vi "SafeBiasSet.vi"(0 "Application ref in":refnum<vi>, 1 "Bias (V)":sgl=-2.0 format="%_5p", 2 "Ramp":bool=TRUE, 3 "error in (no error)":errorcluster, 4 "milliseconds to wait":u32=2) -> (7 "Application ref out":refnum<vi>, 10 "Error out":errorcluster)   [LabVIEW 2021]
uses:
  <userlib>/Nanonis Prog Interface V5/Nanonis Prog Interface.lvlib
panel:
  in  "Bias (V) StepSize":sgl=0.05 format="%_5p"
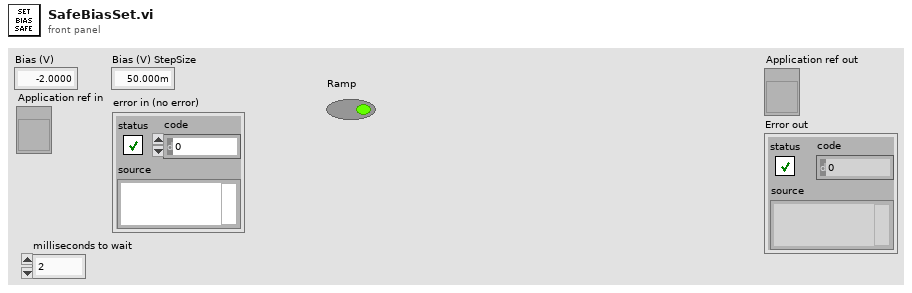
[diagram p1: front panel]
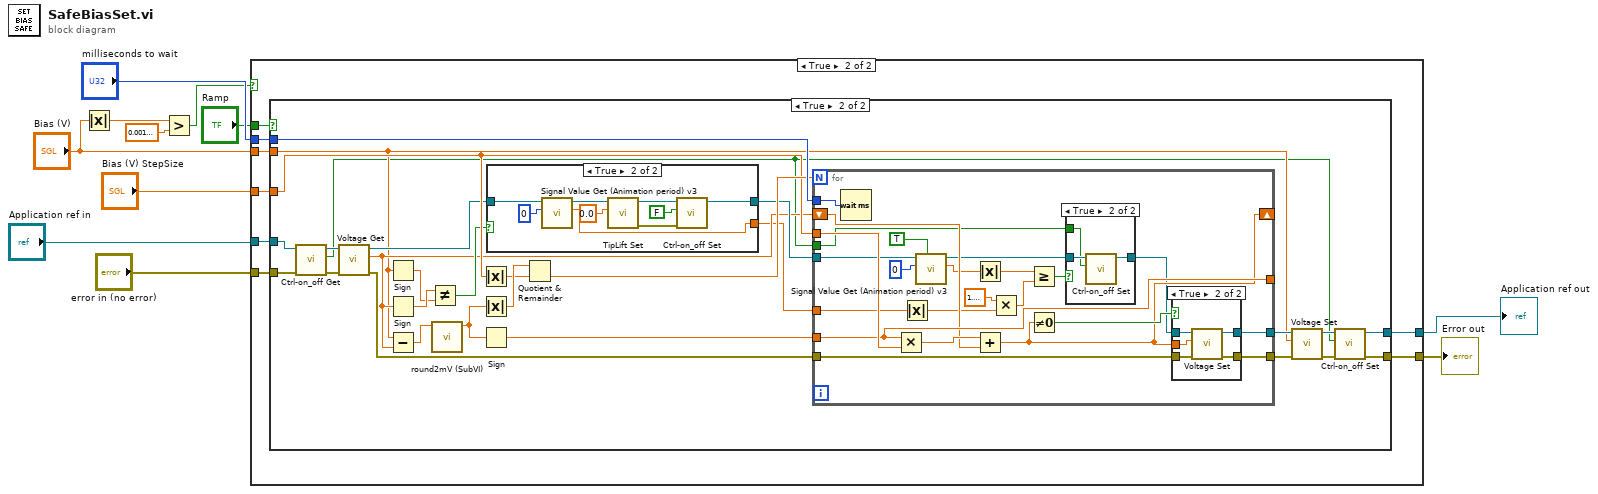
[diagram p0: block diagram]
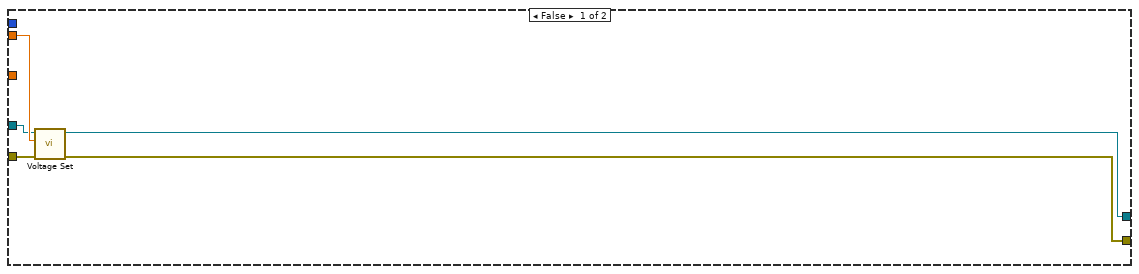
[diagram p3: hidden frame]
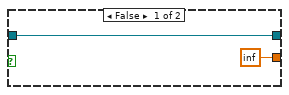
[diagram p4: hidden frame]
diagram:
  n1 = Absolute Value(x="Bias (V)") -> (abs(x)=w4:sgl)
  n2 = Greater?(x=w4, y=sgl 0.001) -> (0:w8:bool)
  n3 = case shown="True" w8 {
    tunnel: "Application ref in" -> [w13 w19]
    tunnel: "Bias (V)" -> [_ w15]
    tunnel: "error in (no error)" -> [w12 w16]
    tunnel: [w12 w17] -> w10
    tunnel: "milliseconds to wait" -> [_ w21]
    tunnel: "Bias (V) StepSize" -> [_ w20]
    tunnel: [w13 w18] -> w3
    tunnel: "Ramp" -> [_ w14]
    frame False {
    }
    frame True {
      n4 = case shown="True" w14 {
        tunnel: w21 -> [_ w54]
        tunnel: w20 -> [_ w46]
        tunnel: w19 -> [w25 w43]
        tunnel: [w23 w37] -> w18
        tunnel: [w22 w36] -> w17
        tunnel: w16 -> [w24 w35]
        tunnel: w15 -> [w26 w30]
        frame False {
          n5 = call <userlib>:"Voltage Set.vi"("Error in (no error)"=w24, "Bias (V)"=w26, "Application ref in"=w25) -> ("Error out"=w22:errorcluster, "Application ref out"=w23:refnum<vi>)  [unwired: 7 in]
        }
        frame True {
          n6 = call <userlib>:"Ctrl-on_off Get.vi"("error in (no error)"=w35, "Application ref in"=w43) -> ("error out"=w34:errorcluster, "Z-Controller on/off status"=w27:bool, "Application ref out"=w42:refnum<vi>)  [unwired: 7 in]
          n7 = call <userlib>:"Voltage Get.vi"("error in (no error)"=w34, "Application ref in"=w42) -> ("error out"=w53:errorcluster, "Bias (V)"=w31:sgl, "Application ref out"=w41:refnum<vi>)  [unwired: 7 in]
          n8 = Sign(1:w30) -> (0:w29:sgl)
          n9 = Sign(1:w31) -> (0:w32:sgl)
          n10 = Subtract(x=w30, y=w31) -> (x-y=w51:sgl)
          n11 = Not Equal?(x=w32, y=w29) -> (x != y?=w33:bool)
          n12 = call "round2mV (SubVI).vi"("Numeric in"=w51) -> ("Numeric out"=w48:dbl)  [unwired: 10 in]
          n13 = Absolute Value(x=w46) -> (abs(x)=w47:sgl)
          n14 = Absolute Value(x=w48) -> (abs(x)=w49:dbl)
          n15 = Sign(1:w48) -> (0:w52:dbl)
          n16 = case shown="True" w33 {
            tunnel: w41 -> [w56 w60]
            tunnel: [w56 w61] -> w40
            tunnel: [sgl inf ("Signal value") w57] -> w28
            frame False {
            }
            frame True {
              n17 = call <userlib>:"Signal Value Get (Animation period) v3.vi"("Signal index (0-127)"=i8 0 ("Signal index (0-79)"), "Application ref in"=w60) -> ("Signal value"=w57:sgl, "Application ref out"=w59:refnum<vi>)  [unwired: 6 in, 1 out]
              n18 = call <userlib>:"TipLift Set.vi"("TipLift (m)"=sgl 0.0, "Application ref in"=w59) -> ("error out"=w65:errorcluster, "Application ref out"=w64:refnum<vi>)  [unwired: 8 in]
              n19 = call <userlib>:"Ctrl-on_off Set.vi"("error in (no error)"=w65, "Z Controller ON/OFF"=FALSE, "Application ref in"=w64) -> ("Application ref out"=w61:refnum<vi>)  [unwired: 7 in, 1 out]
            }
          }
          n20 = Quotient & Remainder(x=w49, y=w47) -> (floor(x/y)=w50:dbl)  [unwired: 1 out]
          n21 = for {
            N: w50 -> [_]
            tunnel: w40 -> [w78]
            tunnel: [w88] -> w45
            tunnel: w53 -> [w82]
            tunnel: [w87] -> w44
            tunnel: w54 -> [w86]
            tunnel: w46 -> [w85]
            tunnel: w52 -> [w83]
            tunnel: [w83] -> _
            shift-right: [w79] -> _
            shift-left: w31 -> [w81]
            tunnel: w28 -> [w75]
            tunnel: w27 -> [w69]
            n22 = Wait (ms)(milliseconds to wait=w86) -> ()  [unwired: 1 out]
            n23 = Multiply(x=w83, y=w85) -> (x*y=w84:dbl)
            n24 = Absolute Value(x=w75) -> (abs(x)=w74:sgl)
            n25 = call <userlib>:"Signal Value Get (Animation period) v3.vi"("Wait for newest data (F=False)"=TRUE, "Signal index (0-127)"=i8 0 ("Signal index (0-79)"), "Application ref in"=w78) -> ("Signal value"=w76:sgl, "Application ref out"=w71:refnum<vi>)  [unwired: 5 in, 1 out]
            n26 = Absolute Value(x=w76) -> (abs(x)=w73:sgl)
            n27 = Add(x=w84, y=w81) -> (x+y=w79:dbl)
            n28 = Multiply(x=sgl 1.1, y=w74) -> (x*y=w67:sgl)
            n29 = Greater Or Equal?(x=w73, y=w67) -> (x >= y?=w72:bool)
            n30 = Not Equal To 0?(x=w79) -> (x != 0?=w80:bool)
            n31 = case shown="True" w72 {
              tunnel: w71 -> [w89 w92]
              tunnel: [w89 w91] -> w70
              tunnel: w69 -> [_ w90]
              frame False {
              }
              frame True {
                n32 = call <userlib>:"Ctrl-on_off Set.vi"("Z Controller ON/OFF"=w90, "Application ref in"=w92) -> ("Application ref out"=w91:refnum<vi>)  [unwired: 8 in, 1 out]
              }
            }
            n33 = case shown="True" w80 {
              tunnel: [w94 w99] -> w88
              tunnel: [w93 w98] -> w87
              tunnel: w82 -> [w93 w97]
              tunnel: w70 -> [w94 w96]
              tunnel: w79 -> [_ w95]
              frame False {
              }
              frame True {
                n34 = call <userlib>:"Voltage Set.vi"("Error in (no error)"=w97, "Bias (V)"=w95, "Application ref in"=w96) -> ("Error out"=w98:errorcluster, "Application ref out"=w99:refnum<vi>)  [unwired: 7 in]
              }
            }
          }
          n35 = call <userlib>:"Voltage Set.vi"("Error in (no error)"=w44, "Bias (V)"=w30, "Application ref in"=w45) -> ("Error out"=w38:errorcluster, "Application ref out"=w39:refnum<vi>)  [unwired: 7 in]
          n36 = call <userlib>:"Ctrl-on_off Set.vi"("error in (no error)"=w38, "Z Controller ON/OFF"=w27, "Application ref in"=w39) -> ("error out"=w36:errorcluster, "Application ref out"=w37:refnum<vi>)  [unwired: 7 in]
        }
      }
    }
  }
  "Application ref out" <- w3
  "Error out" <- w10
